vi "SS_b4Trigger.vi"(6 "Main Cluster IN":T1, 8 "Error In":errorcluster, 11 "Info In":string="\nWaiting for TimerScope Trigger\n- IN: SS TimerScope Trigger\n- OUT: SET SS ThermoRec Received Trigger\nPulse Number is 231123\nPulse Type is 4\n\nDuration (s) is  2.000000\nDelay (s)  is  1.000000\nScan Period (ms) is  15\nNumber of Samples is  134\n\nDelay Started\nDelay Complete\nExternal Measurement of Delay (s): 1.000000\nACQUIRING DATA") -> (0 "Error Out":errorcluster, 3 "Info Out":string="\nWaiting for TimerScope Trigger\n- IN: SS TimerScope Trigger\n- OUT: SET SS ThermoRec Received Trigger\nPulse Number is 231123\nPulse Type is 4\n\nDuration (s) is  2.000000\nDelay (s)  is  1.000000\nScan Period (ms) is  15\nNumber of Samples is  134\n\nDelay Started\nDelay Complete\nExternal Measurement of Delay (s): 1.000000\nACQUIRING DATA", 4 "Main Cluster OUT":T1)   [LabVIEW 2016]
uses:
  Control/Control_Main.ctl
  Control/Control_ModuleArray.ctl
panel:
  in  "Tab Control":enum32{"IN", "OUT", "SubVI Info"}(tab)
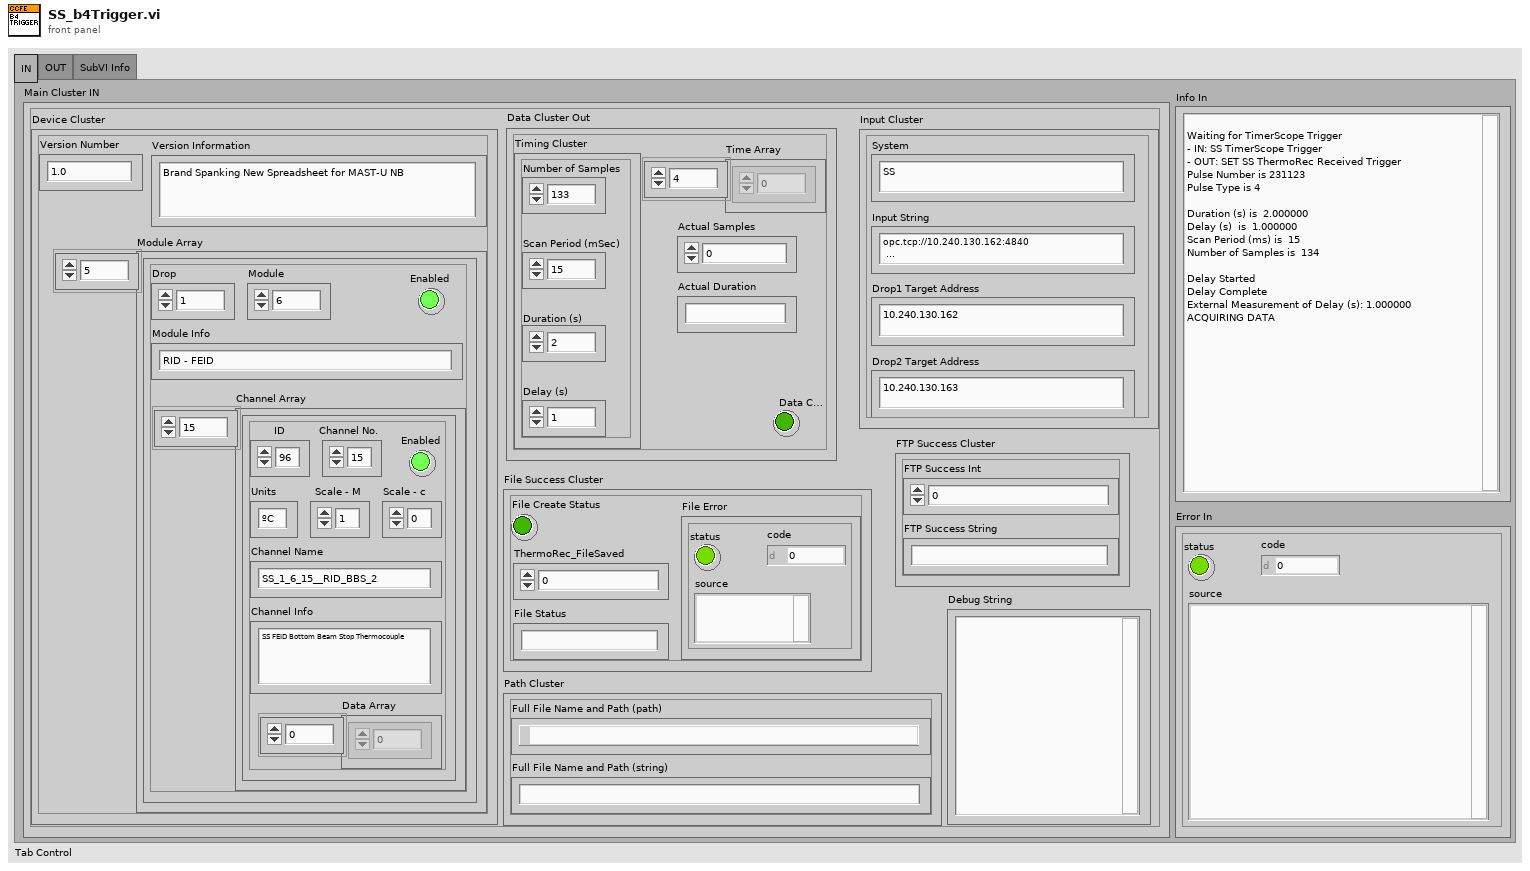
[diagram p1: front panel]
types:
  T1 = typedef "Control_Main.ctl" = cluster{"Device Cluster":cluster{"Module Array":T2, "Version Number":string, "Version Information":string}, "Input Cluster":cluster{"Input String":string, "Drop1 Target Address":string, "Drop2 Target Address":string, "System":string}, "Data Cluster Out":cluster{"Timing Cluster":cluster{"Number of Samples":i32, "Scan Period (mSec)":u32, "Duration (s)":dbl, "Delay (s)":dbl}, "Time Array":dbl[], "Actual Samples":i32, "Actual Duration":string, "Data Collection Error":bool}, "Path Cluster":cluster{"Full File Name and Path (path)":path, "Full File Name and Path (string)":string}, "File Success Cluster":cluster{"ThermoRec_FileSaved":i32, "File Create Status":bool, "File Error":errorcluster, "File Status":string}, "FTP Success Cluster":cluster{"FTP Success Int":i32, "FTP Success String":string}, "Debug String":string}
  T2 = typedef "Control_ModuleArray.ctl" = cluster{"Drop":i32, "Module":i32, "Module Info":string, "Enabled":bool, "Channel Array":cluster{"ID":i32, "Channel No.":i32, "Enabled":bool, "Channel Name":string, "Channel Info":string, "Units":string, "Scale - M":dbl, "Scale - c":dbl, "Data Array":dbl[]}[]}[]
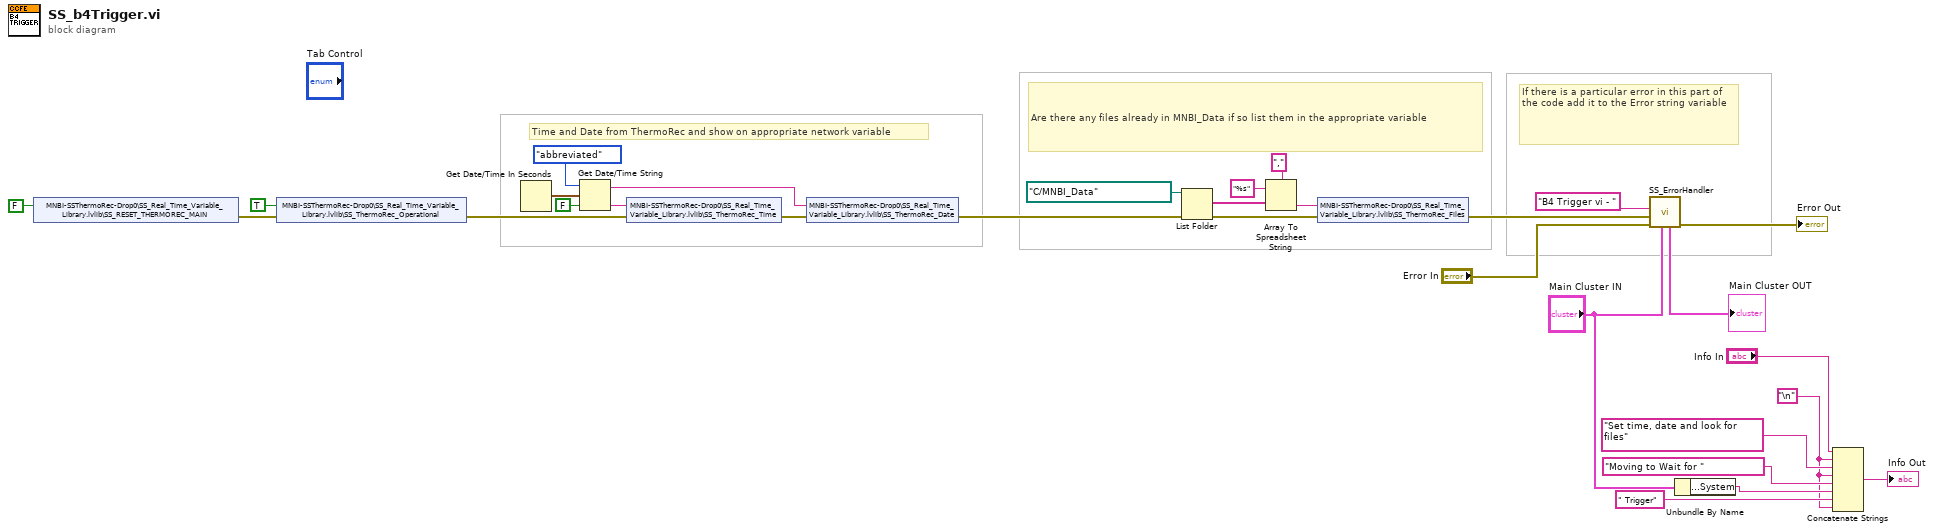
[diagram p0: block diagram]
diagram:
  w1 = "\n"
  # "If there is a particular error in this part of the code add it to the Error string variable"
  # "Are there any files already in MNBI_Data if so list them in the appropriate variable"
  # "Time and Date from ThermoRec and show on appropriate network variable"
  n1 = shared-variable "MNBI-SSThermoRec-Drop0\\SS_Real_Time_Variable_Library.lvlib\\SS_RESET_THERMOREC_MAIN"(FALSE ("SS_RESET_THERMOREC_MAIN")) -> (error out=w16:errorcluster)  [unwired: 1 in]
  n2 = shared-variable "MNBI-SSThermoRec-Drop0\\SS_Real_Time_Variable_Library.lvlib\\SS_ThermoRec_Operational"(TRUE ("SS_RESET_THERMOREC_MAIN"), error in=w16) -> (error out=w18:errorcluster)
  n3 = Get Date/Time In Seconds() -> (seconds since 1Jan1904=w28:timestamp)
  n4 = Get Date/Time String(date format (0)=enum16{"short", "long", "abbreviated"}."abbreviated", seconds (now)=w28, want seconds? (F)=FALSE) -> (date string=w25:string, time string=w24:string)
  n5 = shared-variable "MNBI-SSThermoRec-Drop0\\SS_Real_Time_Variable_Library.lvlib\\SS_ThermoRec_Time"(w24, error in=w18) -> (error out=w29:errorcluster)
  n6 = shared-variable "MNBI-SSThermoRec-Drop0\\SS_Real_Time_Variable_Library.lvlib\\SS_ThermoRec_Date"(w25, error in=w29) -> (error out=w9:errorcluster)
  n7 = List Folder(path=path "C:/MNBI_Data", error in=w9) -> (filenames=w21:string[], error out=w10:errorcluster)  [unwired: 2 in, 2 out]
  n8 = Array To Spreadsheet String(delimiter (Tab)=",", array=w21, 3:"%s" ("delimiter (Tab)")) -> (spreadsheet string=w20:string)
  n9 = shared-variable "MNBI-SSThermoRec-Drop0\\SS_Real_Time_Variable_Library.lvlib\\SS_ThermoRec_Files"(w20, error in=w10) -> (error out=w13:errorcluster)
  n10 = call "SS_ErrorHandler.vi"("Main Cluster IN"="Main Cluster IN", "Error In"="Error In", "SubVI Error"=w13, "SubVI Name"="B4 Trigger vi - ") -> ("Error Out"=→"Error Out":errorcluster, "Main Cluster OUT"=→"Main Cluster OUT":T1)  [unwired: 5 in, 1 out]
  n11 = Unbundle By Name("Main Cluster IN") -> ("Input Cluster.System"=w6:string)
  n12 = Concatenate Strings("Info In", w1, "Set time, date and look for files" ("string"), w1, "Moving to Wait for " ("string"), w6, " Trigger" ("string"), w1) -> (→"Info Out":string)
